vi "CRYView Model Message.vi"(8 "nData":i32, 9 "sData":string, 10 "sOption":string, 11 "sMsgData":string) -> (0 "nData_Out":i32, 1 "sData_Out":string, 3 "cView_Out":T1)   [LabVIEW 2013]
uses:
  CRYNew View Global.vi
  SubVI/CRYData View Global.vi
  CRYView Global.vi
  CRYCurveLibrary/Global/CRYCurve Library Global.vi
  CRYProject/CRYProject Editor Global.vi
panel:
  in  "Resize_Panels":bool
  out "Bar_shadow":bool
  in  "splitter_down_flag":bool=TRUE
  in  "sMsgAction":string
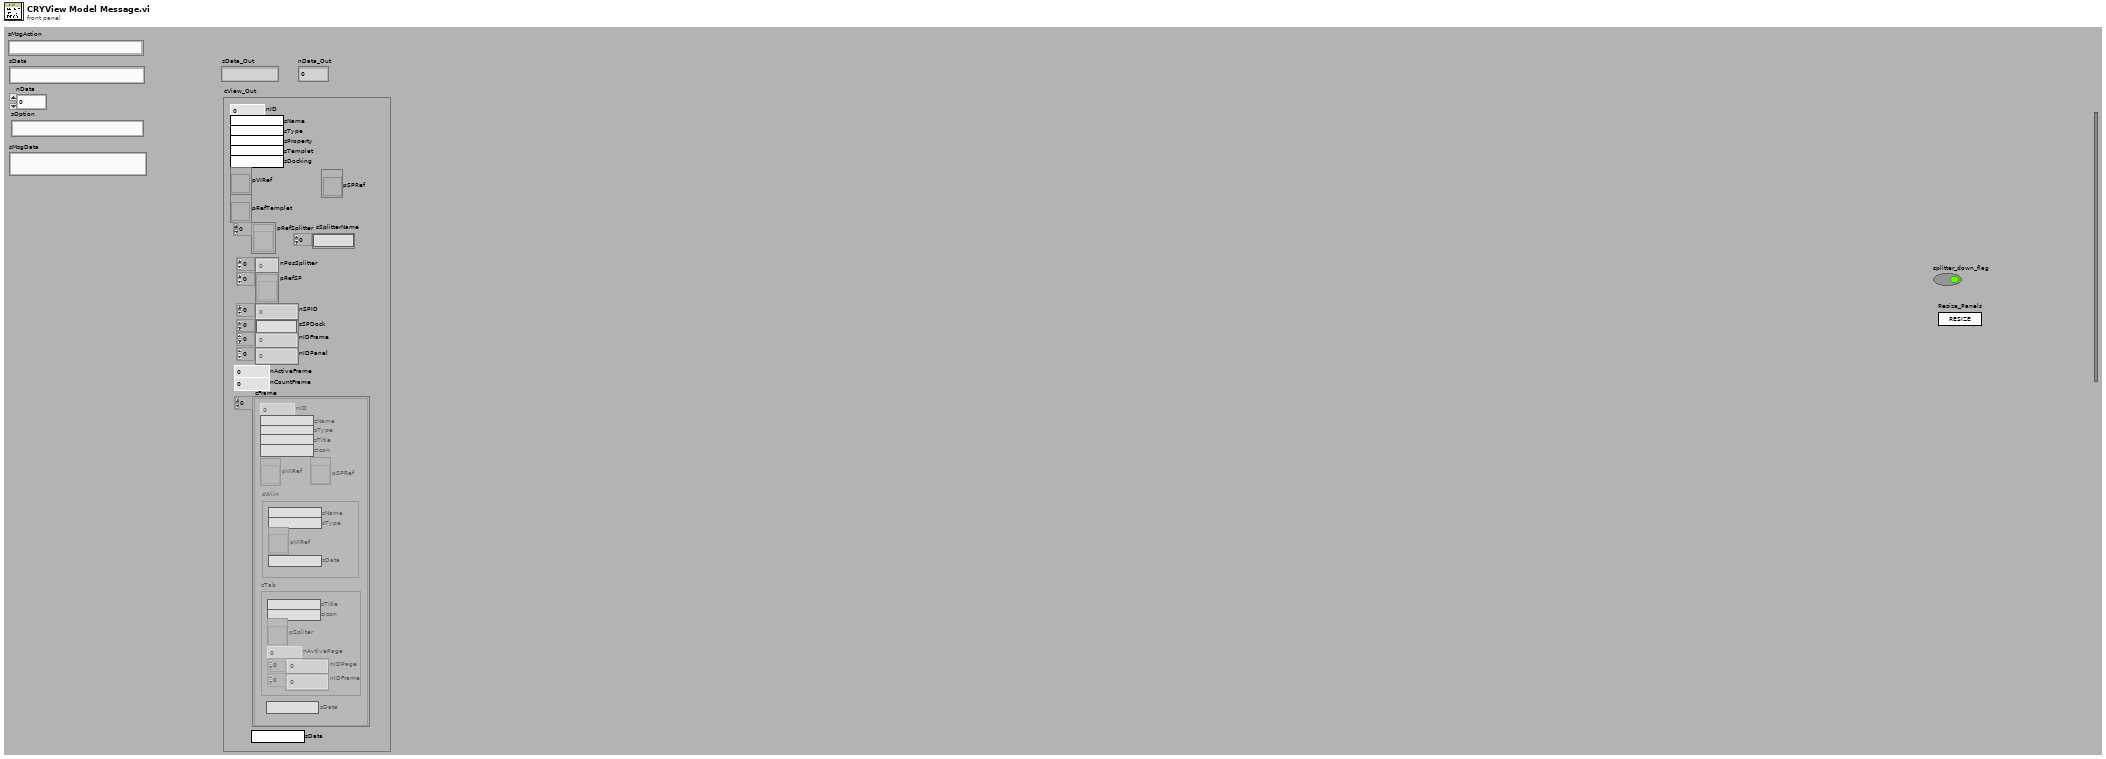
[diagram p1: front panel]
types:
  T1 = cluster{"nID":i32, "sName":string, "sType":string, "sProperty":string, "sTemplet":string, "sDocking":string, "pVIRef":refnum<vi>, "pSPRef":refnum<vi>, "pRefTemplet":refnum<vi>, "pRefSplitter":refnum<vi>[], "nPosSplitter":i32[], "pRefSP":refnum<vi>[], "nSPID":i32[], "sSPDock":string[], "nIDFrame":i32[], "nIDPanel":i32[], "nActiveFrame":i32, "nCountFrame":i32, "cFrame":cluster{"nID":i32, "sName":string, "sType":string, "sTitle":string, "sIcon":string, "pVIRef":refnum<vi>, "pSPRef":refnum<vi>, "cWiin":cluster{"sName":string, "sType":string, "pVIRef":refnum<vi>, "sData":string}, "cTab":cluster{"sTitle":string, "sIcon":string, "pSpliter":refnum<vi>, "nAvtivePage":i32, "nIDPage":i32[], "nIDFrame":i32[]}, "sData":string}[], "sData":string, "sSplitterName":string[]}
  T2 = typedef "Graph Main Info Cluster.ctl" = cluster{"Selected_BarIdx":i32, "Selected_PanelIdx":i32, "Graph Main VIRef":refnum<vi>, "ToolBarClick":bool, "Spliter Ref Array":refnum<vi>[], "Panel Ref Array":refnum<vi>[], "Spliter_matrix":i32[][], "Panel_matrix":i32[][], "child_spliterIdx_matrix":i32[][], "split_pos_matrix":i32[][], "Title State":bool, "sQueueName":string, "Frame nID":i32, "Graph VIRef Array":cluster{"Graph VIRef":refnum<vi>, "Panel Idx":i32, "Frame VIRef":refnum<vi>, "Icon Ring":i32, "Graph Type":string}[], "View Type":string}
  T3 = cluster{"Graph VIRef":refnum<vi>, "Panel Idx":i32, "Frame VIRef":refnum<vi>, "Icon Ring":i32, "Graph Type":string}[]
  T4 = cluster{"EventName":string, "Arg1":string, "Numeric":u16, "Numeric 2":u16, "AddSteps ":refnum<vi>, "Arg1 2":string, "Arg1 3":string, "Boolean":bool}
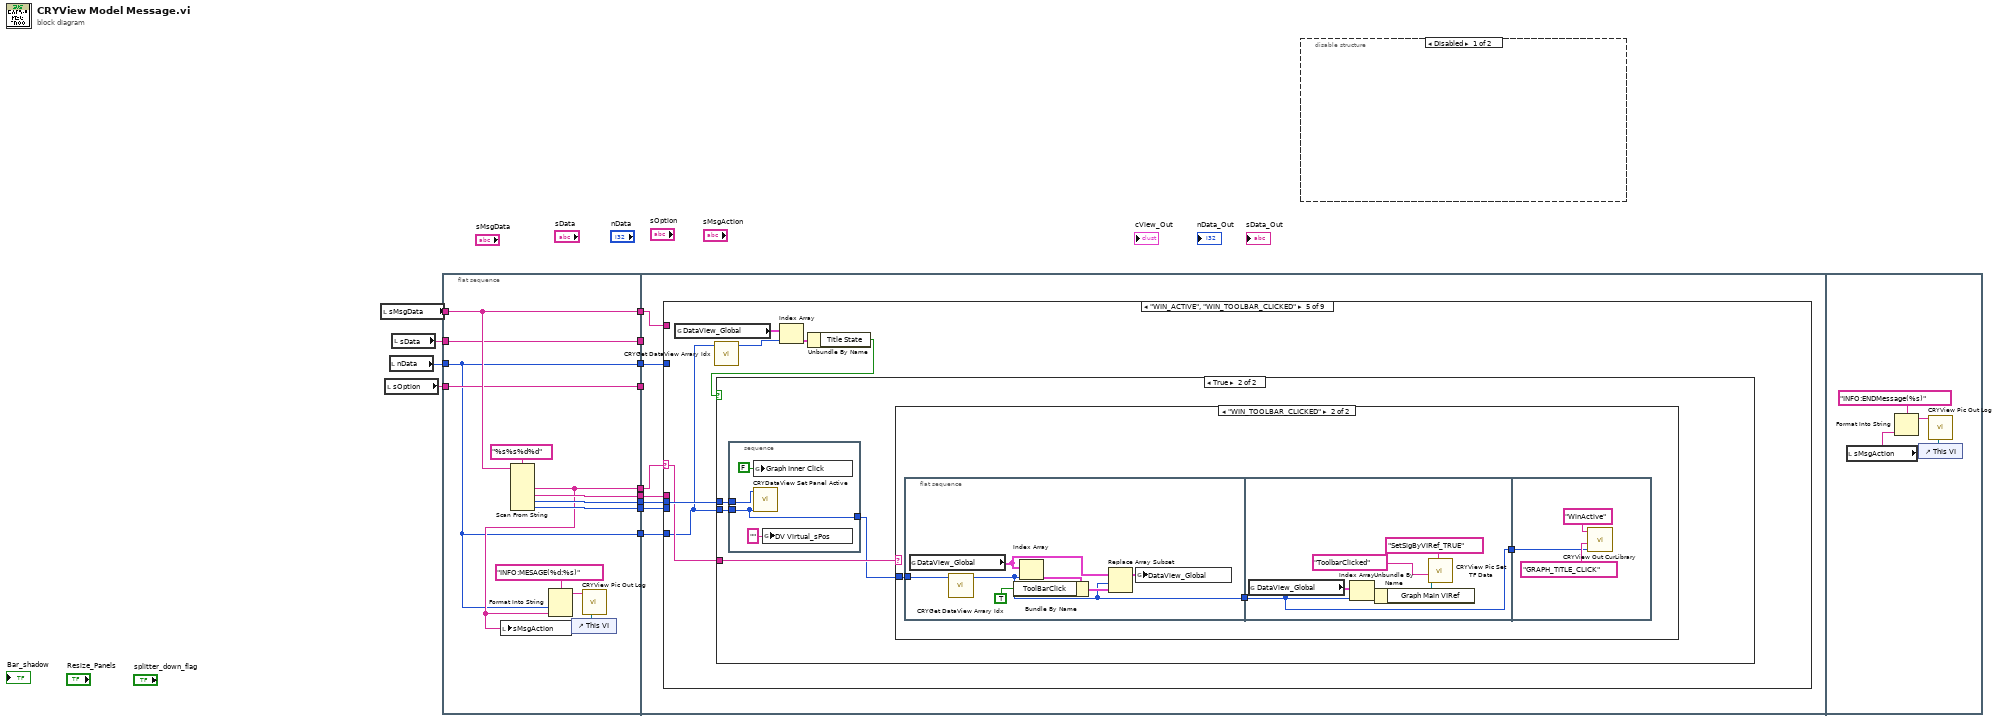
[diagram p0: block diagram]
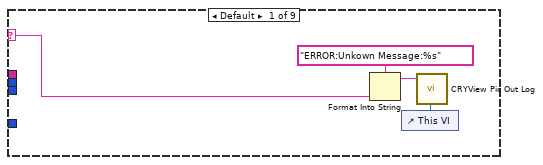
[diagram p3: hidden frame]
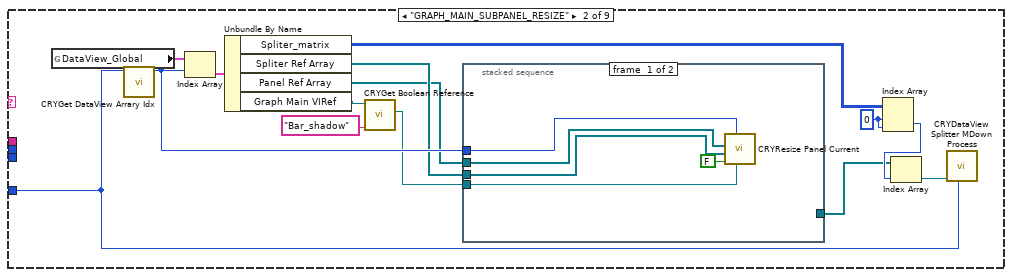
[diagram p4: hidden frame]
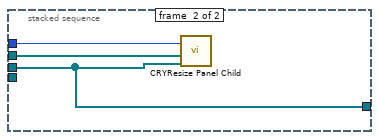
[diagram p5: hidden frame]
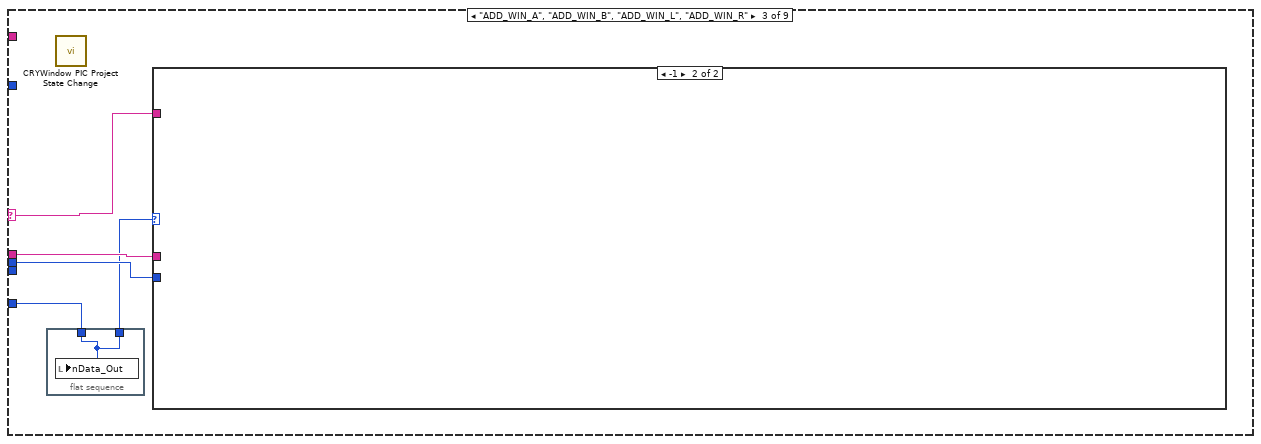
[diagram p6: hidden frame]
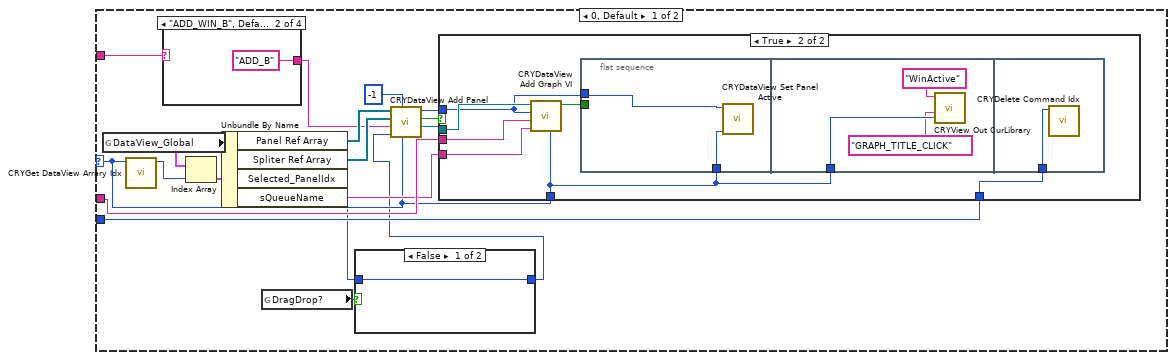
[diagram p7: hidden frame]
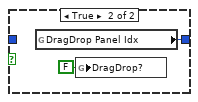
[diagram p8: hidden frame]
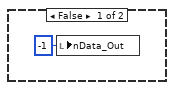
[diagram p9: hidden frame]
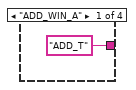
[diagram p10: hidden frame]
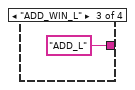
[diagram p11: hidden frame]
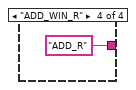
[diagram p12: hidden frame]
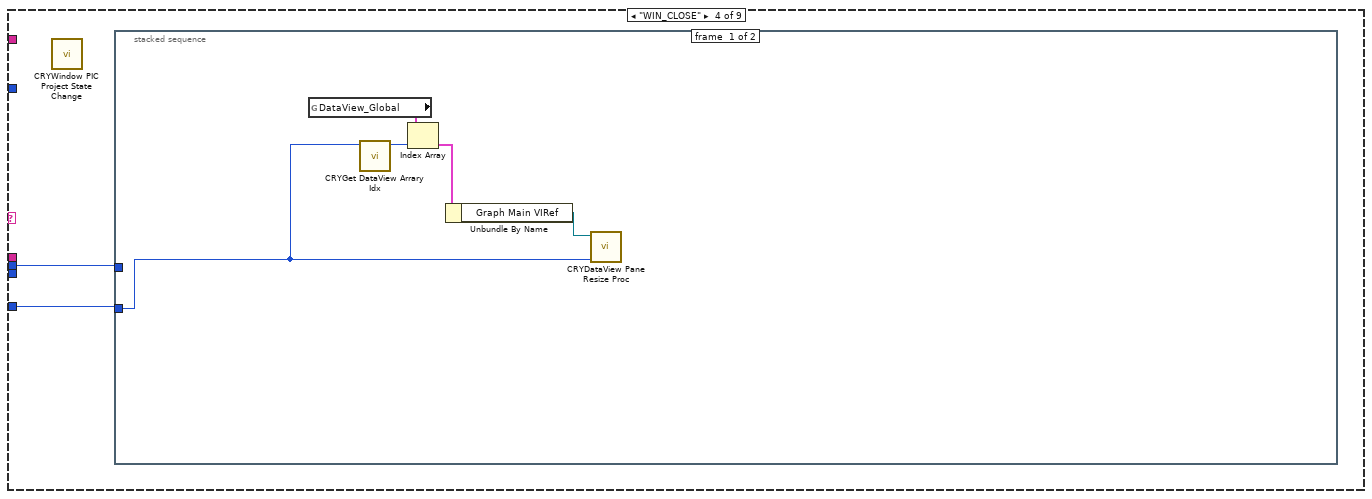
[diagram p13: hidden frame]
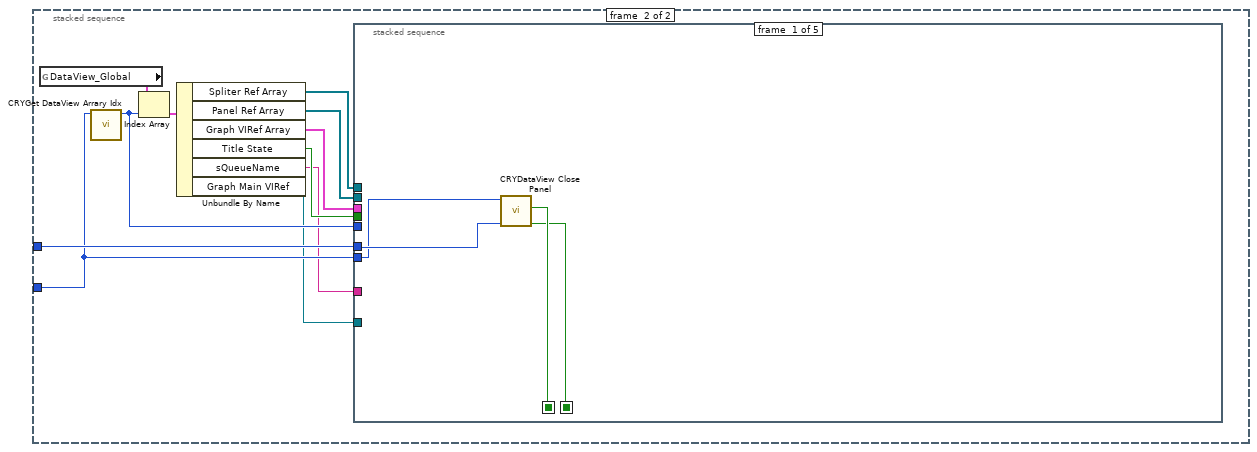
[diagram p14: hidden frame]
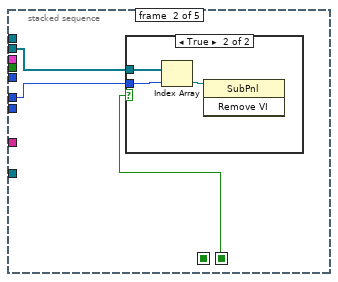
[diagram p15: hidden frame]
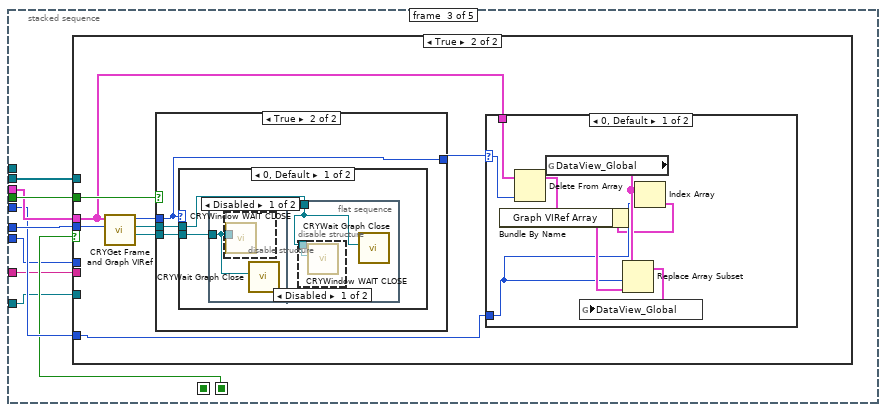
[diagram p17: hidden frame]
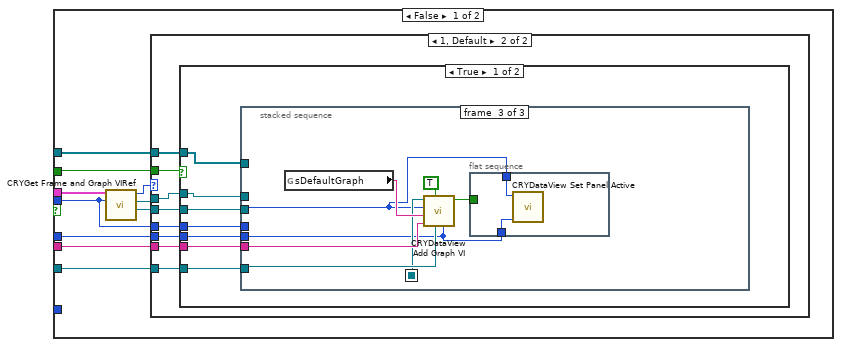
[diagram p18: hidden frame]
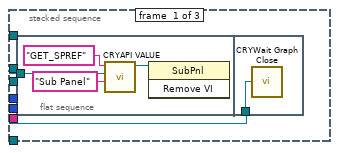
[diagram p20: hidden frame]
diagram:
  n1 = local read "sMsgData"() -> (w13:string)
  n2 = local read "sOption"() -> (w11:string)
  n3 = local read "nData"() -> (w12:i32)
  n4 = local read "sData"() -> (w5:string)
  n5 = flat-sequence {
    tunnel: w13 -> [w24]
    tunnel: w12 -> [w14]
    tunnel: w11 -> [w19]
    tunnel: [w24] -> w10
    tunnel: [w15] -> w9
    tunnel: [w23] -> w8
    tunnel: [w21] -> w7
    tunnel: [w22] -> w6
    tunnel: w5 -> [w20]
    tunnel: [w20] -> w4
    tunnel: [w14] -> w3
    tunnel: [w19] -> w2
    tunnel: [w14] -> w1
    tunnel: w10 -> [w28]
    tunnel: w9 -> [w32]
    tunnel: w8 -> [w31]
    tunnel: w7 -> [w30]
    tunnel: w6 -> [w29]
    tunnel: w4 -> [_]
    tunnel: w3 -> [w27]
    tunnel: w2 -> [_]
    tunnel: w1 -> [w26]
    frame #0 {
      n6 = Scan From String(format string="%s%s%d%d", input string=w24) -> (output 1=w15:string, output 2=w23:string, output 3=w21:i32, output 4=w22:i32)  [unwired: 2 in, 7 out]
      n7 = local write "sMsgAction"(w15) -> ()
      n8 = Format Into String(format string="INFO:MESAGE(%d:%s)", w14, w15) -> (resulting string=w17:string)  [unwired: 2 in, 1 out]
      n9 = control-ref of="This VI"() -> (w18:refnum<vi>)
      n10 = call "CRYView Pic Out Log.vi"("vi reference"=w18, "sData"=w17) -> ()  [unwired: 10 in]
    }
    frame #1 {
      n11 = case shown="\"WIN_ACTIVE\", \"WIN_TOOLBAR_CLICKED\"" w32 {
        selector: w32 -> [w34 _ w62 _ w282 _ _ w320 _]
        tunnel: w31 -> [_ _ w63 _ _ _ _ _ w328]
        tunnel: w30 -> [_ _ w61 w105 w283 _ _ w322 w332]
        tunnel: w29 -> [_ _ _ _ _ _ _ _ _]
        tunnel: w28 -> [_ _ _ _ _ _ _ w319 _]
        tunnel: w27 -> [_ _ _ _ _ _ _ _ w331]
        tunnel: w26 -> [_ w37 w60 w104 w279 _ _ w317 _]
        frame Default {
          n12 = Format Into String(format string="ERROR:Unkown Message:%s", w34) -> (resulting string=w33:string)  [unwired: 2 in, 1 out]
          n13 = control-ref of="This VI"() -> (w36:refnum<vi>)
          n14 = call "CRYView Pic Out Log.vi"("vi reference"=w36, "sData"=w33) -> ()  [unwired: 10 in]
        }
        frame "GRAPH_MAIN_SUBPANEL_RESIZE" {
          w48 = 0 ("index (row)")
          n15 = global read "CRYNew View Global.vi" "DataView_Global"() -> (w41:T2[])
          n16 = call "CRYGet DataView Arrary Idx.vi"("DataView Idx In"=w37) -> ("DataView Arrary Idx out"=w50:i32)  [unwired: 10 in]
          n17 = Index Array(array=w41, index=w50) -> (element=w42:T2)
          n18 = Unbundle By Name(w42) -> ("Spliter_matrix"=w46:i32[][], "Spliter Ref Array"=w44:refnum<vi>[], "Panel Ref Array"=w43:refnum<vi>[], "Graph Main VIRef"=w40:refnum<vi>)
          n19 = call "CRYGet Boolean Reference.vi"("Label Name"="Bar_shadow", "VI Refnum"=w40) -> ("Boolean Ref"=w38:refnum<vi>)  [unwired: 7 in, 2 out]
          n20 = stacked-sequence {
            tunnel: w44 -> [w54 w56]
            tunnel: w43 -> [w55 w58]
            tunnel: w50 -> [w53 w57]
            tunnel: [_ w56] -> w45
            tunnel: w38 -> [w52 _]
            frame #0 {
              n21 = call "CRYResize Panel Current.vi"("Bar_shadow"=w52, "DataView Array Idx"=w53, "close_panel"=FALSE, "spliter array"=w54, "SubPanel array"=w55) -> ()  [unwired: 7 in]
            }
            frame #1 {
              n22 = call "CRYResize Panel Child.vi"("spliter array"=w56, "SubPanel array"=w58, "DataView Array Idx"=w57) -> ()  [unwired: 9 in]
            }
          }
          n23 = Index Array(array=w46, index (row)=w48, index (col)=w48) -> (element=w49:i32)
          n24 = Index Array(array=w45, index=w49) -> (element=w47:refnum<vi>)
          n25 = call "CRYDataView Splitter MDown Process.vi"("DataView Index"=w37, "Selected Spliter Ref"=w47) -> ()  [unwired: 9 in, 1 out]
        }
        frame "ADD_WIN_A", "ADD_WIN_B", "ADD_WIN_L", "ADD_WIN_R" {
          n26 = flat-sequence {
            tunnel: w60 -> [w64]
            tunnel: [w64] -> w59
            frame #0 {
              n27 = local write "nData_Out"(w64) -> ()
            }
          }
          n28 = call "CRYWindow PIC Project State Change.vi"() -> ()  [unwired: 12 in]
          n29 = case shown="-1" w59 {
            selector: w59 -> [w69 _]
            tunnel: w62 -> [w79 _]
            tunnel: w63 -> [w71 _]
            tunnel: w61 -> [w68 _]
            frame 0, Default {
              n30 = global read "CRYNew View Global.vi" "DataView_Global"() -> (w82:T2[])
              n31 = call "CRYGet DataView Arrary Idx.vi"("DataView Idx In"=w69) -> ("DataView Arrary Idx out"=w81:i32)  [unwired: 10 in]
              n32 = case shown="\"ADD_WIN_B\", Default" w79 {
                tunnel: ["ADD_T" ("input 1") "ADD_B" ("input 1") "ADD_L" ("input 1") "ADD_R" ("input 1")] -> w75
                frame "ADD_WIN_A" {
                }
                frame "ADD_WIN_B", Default {
                }
                frame "ADD_WIN_L" {
                }
                frame "ADD_WIN_R" {
                }
              }
              n33 = Index Array(array=w82, index=w81) -> (element=w80:T2)
              n34 = Unbundle By Name(w80) -> ("Panel Ref Array"=w77:refnum<vi>[], "Spliter Ref Array"=w76:refnum<vi>[], "Selected_PanelIdx"=w66:i32, "sQueueName"=w70:string)
              n35 = global read "CRYData View Global.vi" "DragDrop?"() -> (w67:bool)
              n36 = case shown="False" w67 {
                tunnel: [w83 w84] -> w65
                tunnel: w66 -> [w83 _]
                frame False {
                }
                frame True {
                  n37 = global read "CRYData View Global.vi" "DragDrop Panel Idx"() -> (w84:i32)
                  n38 = global write "CRYData View Global.vi" "DragDrop?"(FALSE ("DragDrop?")) -> ()
                }
              }
              n39 = call "CRYDataView Add Panel.vi"("DataView Index"=w69, "panel_index"=-1, "Selected Panel Idx"=w65, "SAdd_Pos"=w75, "spliter array"=w76, "SubPanel array"=w77) -> ("Panel Ref"=w72:refnum<vi>, "bResult"=w74:bool, "panel_index_out"=w73:i32)  [unwired: 3 in]
              n40 = case shown="True" w74 {
                tunnel: w73 -> [_ w90]
                tunnel: w72 -> [_ w93]
                tunnel: w71 -> [_ w92]
                tunnel: w70 -> [_ w91]
                tunnel: w68 -> [_ w88]
                tunnel: w69 -> [_ w87]
                frame False {
                  n41 = local write "nData_Out"(-1 ("nData_Out")) -> ()
                }
                frame True {
                  n42 = call "CRYDataView Add Graph VI.vi"("DataView Idx"=w87, "Queue Name"=w91, "GraphType"=w92, "panel_index"=w90, "Panel Ref In"=w93) -> ("bResult"=w89:bool)  [unwired: 6 in]
                  n43 = flat-sequence {
                    tunnel: w90 -> [w95]
                    tunnel: w89 -> [_]
                    tunnel: w87 -> [w94]
                    tunnel: w87 -> [w98]
                    tunnel: w88 -> [w99]
                    frame #0 {
                      n44 = call "CRYDataView Set Panel Active.vi"("DataView Index"=w94, "Selected Panel Idx In"=w95) -> ()  [unwired: 10 in]
                    }
                    frame #1 {
                      n45 = call "CRYView Out CurLibrary.vi"("DataView Idx"=w98, "sData"="GRAPH_TITLE_CLICK", "sAction"="WinActive") -> ()  [unwired: 7 in, 2 out]
                    }
                    frame #2 {
                      n46 = call "CRYDelete Command Idx.vi"("Command Idx In"=w99) -> ()  [unwired: 11 in]
                    }
                  }
                }
              }
            }
            frame -1 {
            }
          }
        }
        frame "WIN_CLOSE" {
          n47 = call "CRYWindow PIC Project State Change.vi"() -> ()  [unwired: 12 in]
          n48 = stacked-sequence {
            tunnel: w105 -> [_ w121]
            tunnel: w104 -> [w110 w120]
            frame #0 {
              n49 = global read "CRYNew View Global.vi" "DataView_Global"() -> (w109:T2[])
              n50 = call "CRYGet DataView Arrary Idx.vi"("DataView Idx In"=w110) -> ("DataView Arrary Idx out"=w108:i32)  [unwired: 10 in]
              n51 = Index Array(array=w109, index=w108) -> (element=w107:T2)
              n52 = Unbundle By Name(w107) -> ("Graph Main VIRef"=w106:refnum<vi>)
              n53 = call "CRYDataView Pane Resize Proc.vi"("DataView Index"=w110, "VI Ref"=w106) -> ()  [unwired: 10 in]
            }
            frame #1 {
              n54 = global read "CRYNew View Global.vi" "DataView_Global"() -> (w119:T2[])
              n55 = call "CRYGet DataView Arrary Idx.vi"("DataView Idx In"=w120) -> ("DataView Arrary Idx out"=w118:i32)  [unwired: 10 in]
              n56 = Index Array(array=w119, index=w118) -> (element=w113:T2)
              n57 = Unbundle By Name(w113) -> ("Spliter Ref Array"=w117:refnum<vi>[], "Panel Ref Array"=w116:refnum<vi>[], "Graph VIRef Array"=w115:T3, "Title State"=w114:bool, "sQueueName"=w112:string, "Graph Main VIRef"=w111:refnum<vi>)
              n58 = stacked-sequence {
                seq-local: [w125 _ _ _ _] -> [_ _ _ w242 _]
                seq-local: [w123 _ _ _ _] -> [_ w128 w136 _ _]
                tunnel: w121 -> [w124 w126 w140 _ w262]
                tunnel: w120 -> [w122 _ w133 w240 w270]
                tunnel: w116 -> [_ w127 w132 w243 _]
                tunnel: w117 -> [_ _ _ w239 _]
                tunnel: w118 -> [_ _ w137 w241 w260]
                tunnel: w115 -> [_ _ w138 _ _]
                tunnel: w114 -> [_ _ w139 _ _]
                tunnel: w112 -> [_ _ w135 _ _]
                tunnel: w111 -> [_ _ w134 _ _]
                frame #0 {
                  n59 = call "CRYDataView Close Panel.vi"("Panel_Idx"=w124, "DataView Index"=w122) -> ("bResult"=w123:bool, "bHaveChild"=w125:bool)  [unwired: 7 in, 1 out]
                }
                frame #1 {
                  n60 = case shown="True" w128 {
                    tunnel: w127 -> [_ w131]
                    tunnel: w126 -> [_ w130]
                    frame False {
                    }
                    frame True {
                      n61 = Index Array(array=w131, index=w130) -> (element=w129:refnum<vi>)
                      n62 = invoke class="SubPnl" method="Remove VI"(reference=w129) -> ()  [unwired: 2 in, 3 out]
                    }
                  }
                }
                frame #2 {
                  n63 = case shown="True" w136 {
                    tunnel: w140 -> [w145 w217]
                    tunnel: w139 -> [w150 w216]
                    tunnel: w138 -> [w149 w211]
                    tunnel: w137 -> [_ w210]
                    tunnel: w135 -> [w146 _]
                    tunnel: w134 -> [w144 _]
                    tunnel: w133 -> [w143 _]
                    tunnel: w132 -> [w142 _]
                    frame False {
                      n64 = call "CRYGet Frame and Graph VIRef.vi"("Panel Idx"=w145, "Graph VIRef Array"=w149) -> ("Graph VIRef"=w148:refnum<vi>, "Frame VIRef"=w147:refnum<vi>, "Graph VIRef Array Index"=w141:i32)  [unwired: 5 in, 2 out]
                      n65 = case shown="1, Default" w141 {
                        tunnel: w150 -> [_ w158]
                        tunnel: w148 -> [_ w157]
                        tunnel: w147 -> [_ w156]
                        tunnel: w146 -> [_ w155]
                        tunnel: w145 -> [_ w154]
                        tunnel: w144 -> [_ w153]
                        tunnel: w143 -> [_ w152]
                        tunnel: w142 -> [_ w151]
                        frame -1 {
                        }
                        frame 1, Default {
                          n66 = case shown="True" w158 {
                            tunnel: w157 -> [w164 w197]
                            tunnel: w156 -> [w165 _]
                            tunnel: w155 -> [w163 w196]
                            tunnel: w154 -> [w162 w195]
                            tunnel: w153 -> [w161 w194]
                            tunnel: w152 -> [w160 w193]
                            tunnel: w151 -> [w159 w192]
                            frame True {
                              n67 = stacked-sequence {
                                seq-local: [_ w173 _] -> [_ _ w185]
                                tunnel: w165 -> [w167 w174 _]
                                tunnel: w164 -> [w166 _ _]
                                tunnel: w163 -> [_ _ w188]
                                tunnel: w162 -> [_ w175 w182]
                                tunnel: w161 -> [_ _ w187]
                                tunnel: w160 -> [_ _ w183]
                                tunnel: w159 -> [_ w176 _]
                                frame #0 {
                                n68 = flat-sequence {
                                tunnel: w167 -> [w169]
                                tunnel: w166 -> [w172]
                                frame #0 {
                                n69 = call "CRYAPI VALUE.vi"("sControlName"="Sub Panel", "pVIRef"=w169, "sAction"="GET_SPREF") -> ("pSPRef"=w168:refnum<vi>)  [unwired: 2 in, 6 out]
                                n70 = invoke class="SubPnl" method="Remove VI"(reference=w168) -> ()  [unwired: 2 in, 3 out]
                                }
                                frame #1 {
                                n71 = call "CRYWait Graph Close.vi"("vi reference"=w172) -> ()  [unwired: 11 in]
                                }
                                }
                                }
                                frame #1 {
                                n72 = flat-sequence {
                                tunnel: w176 -> [w180]
                                tunnel: w175 -> [w179]
                                tunnel: [w177] -> w173
                                tunnel: w174 -> [w181]
                                frame #0 {
                                n73 = Index Array(array=w180, index=w179) -> (element=w178:refnum<vi>)
                                n74 = invoke class="SubPnl" method="Remove VI"(reference=w178) -> (reference out=w177:refnum<vi>)  [unwired: 2 in, 2 out]
                                }
                                frame #1 {
                                n75 = call "CRYWait Graph Close.vi"("vi reference"=w181) -> ()  [unwired: 11 in]
                                }
                                }
                                }
                                frame #2 {
                                n76 = global read "CRYView Global.vi" "sDefaultGraph"() -> (w189:string)
                                n77 = call "CRYDataView Add Graph VI.vi"("DataView Idx"=w183, "Graph Main VIRef In"=w187, "isFirstPanel"=TRUE, "Queue Name"=w188, "GraphType"=w189, "panel_index"=w182, "Panel Ref In"=w185) -> ("bResult"=w184:bool)  [unwired: 4 in]
                                n78 = flat-sequence {
                                tunnel: w183 -> [w191]
                                tunnel: w184 -> [_]
                                tunnel: w182 -> [w190]
                                frame #0 {
                                n79 = call "CRYDataView Set Panel Active.vi"("DataView Index"=w191, "Selected Panel Idx In"=w190) -> ()  [unwired: 10 in]
                                }
                                }
                                }
                              }
                            }
                            frame False {
                              n80 = stacked-sequence {
                                seq-local: [w201 _ _] -> [_ _ w203]
                                tunnel: w197 -> [_ w202 _]
                                tunnel: w196 -> [_ _ w208]
                                tunnel: w195 -> [w199 _ w207]
                                tunnel: w194 -> [_ _ w206]
                                tunnel: w193 -> [_ _ w204]
                                tunnel: w192 -> [w200 _ _]
                                frame #0 {
                                n81 = Index Array(array=w200, index=w199) -> (element=w198:refnum<vi>)
                                n82 = invoke class="SubPnl" method="Remove VI"(reference=w198) -> (reference out=w201:refnum<vi>)  [unwired: 2 in, 2 out]
                                }
                                frame #1 {
                                n83 = call "CRYWait Graph Close.vi"("vi reference"=w202) -> ()  [unwired: 11 in]
                                }
                                frame #2 {
                                n84 = global read "CRYView Global.vi" "sDefaultGraph"() -> (w209:string)
                                n85 = call "CRYDataView Add Graph VI.vi"("DataView Idx"=w204, "Graph Main VIRef In"=w206, "isFirstPanel"=TRUE, "Queue Name"=w208, "GraphType"=w209, "panel_index"=w207, "Panel Ref In"=w203) -> ()  [unwired: 4 in, 1 out]
                                }
                              }
                            }
                          }
                        }
                      }
                    }
                    frame True {
                      n86 = call "CRYGet Frame and Graph VIRef.vi"("Panel Idx"=w217, "Graph VIRef Array"=w211) -> ("Graph VIRef"=w213:refnum<vi>, "Frame VIRef"=w214:refnum<vi>, "Graph VIRef Array Index"=w215:i32)  [unwired: 5 in, 2 out]
                      n87 = case shown="True" w216 {
                        tunnel: w215 -> [w226 w230]
                        tunnel: w214 -> [_ w231]
                        tunnel: w213 -> [w227 w232]
                        tunnel: [w226 w230] -> w212
                        frame False {
                          n88 = case shown="0, Default" w226 {
                            tunnel: w227 -> [w228 _]
                            frame 0, Default {
                              n89 = disable-structure shown="Disabled" {
                                disable-tunnel: w228 -> [w229 _]
                                frame Disabled {
                                n90 = call "CRYWindow WAIT CLOSE.vi"("vi reference"=w229) -> ()  [unwired: 11 in]
                                }
                                frame Enabled {
                                }
                              }
                              n91 = call "CRYWait Graph Close.vi"("vi reference"=w228) -> ()  [unwired: 11 in]
                            }
                            frame -1 {
                            }
                          }
                        }
                        frame True {
                          n92 = case shown="0, Default" w230 {
                            tunnel: w232 -> [w234 _]
                            tunnel: w231 -> [w233 _]
                            frame 0, Default {
                              n93 = flat-sequence {
                                tunnel: w234 -> [w235]
                                tunnel: w233 -> [w237]
                                frame #0 {
                                n94 = disable-structure shown="Disabled" {
                                disable-tunnel: w235 -> [w236 _]
                                frame Disabled {
                                n95 = call "CRYWindow WAIT CLOSE.vi"("vi reference"=w236) -> ()  [unwired: 11 in]
                                }
                                frame Enabled {
                                }
                                }
                                n96 = call "CRYWait Graph Close.vi"("vi reference"=w235) -> ()  [unwired: 11 in]
                                }
                                frame #1 {
                                n97 = disable-structure shown="Disabled" {
                                disable-tunnel: w237 -> [w238 _]
                                frame Disabled {
                                n98 = call "CRYWindow WAIT CLOSE.vi"("vi reference"=w238) -> ()  [unwired: 11 in]
                                }
                                frame Enabled {
                                }
                                }
                                n99 = call "CRYWait Graph Close.vi"("vi reference"=w237) -> ()  [unwired: 11 in]
                                }
                              }
                            }
                            frame -1 {
                            }
                          }
                        }
                      }
                      n100 = case shown="0, Default" w212 {
                        selector: w212 -> [w224 _]
                        tunnel: w211 -> [w225 _]
                        tunnel: w210 -> [w219 _]
                        frame 0, Default {
                          n101 = Delete From Array(array=w225, index=w224) -> (array with subset deleted=w223:T3)  [unwired: 1 in, 1 out]
                          n102 = global read "CRYNew View Global.vi" "DataView_Global"() -> (w220:T2[])
                          n103 = Index Array(array=w220, index=w219) -> (element=w218:T2)
                          n104 = Bundle By Name(cluster=w218, "Graph VIRef Array"=w223) -> (w222:T2)
                          n105 = Replace Array Subset(array=w220, new element=w222, index=w219) -> (w221:T2[])
                          n106 = global write "CRYNew View Global.vi" "DataView_Global"(w221) -> ()
                        }
                        frame -1 {
                        }
                      }
                    }
                  }
                }
                frame #3 {
                  n107 = case shown="True" w242 {
                    tunnel: w243 -> [_ w248]
                    tunnel: w239 -> [_ w247]
                    tunnel: w241 -> [_ w246]
                    tunnel: w240 -> [w244 w245]
                    tunnel: [w244 w245] -> _
                    frame False {
                    }
                    frame True {
                      n108 = flat-sequence {
                        tunnel: w248 -> [w253]
                        tunnel: w247 -> [w252]
                        tunnel: w246 -> [w254]
                        tunnel: [w254] -> w251
                        tunnel: [w253] -> w250
                        tunnel: [w252] -> w249
                        tunnel: w251 -> [w258]
                        tunnel: w250 -> [w257]
                        tunnel: w249 -> [w256]
                        frame #0 {
                          n109 = call "CRYResize Panel Current.vi"("DataView Array Idx"=w254, "close_panel"=TRUE, "spliter array"=w252, "SubPanel array"=w253) -> ()  [unwired: 8 in]
                        }
                        frame #1 {
                          n110 = call "CRYResize Panel Child.vi"("spliter array"=w256, "SubPanel array"=w257, "DataView Array Idx"=w258) -> ()  [unwired: 9 in]
                        }
                      }
                    }
                  }
                }
                frame #4 {
                  # "if delete no actived graph, preview actived Panel index\nif deleted, first index."
                  n111 = global read "CRYNew View Global.vi" "DataView_Global"() -> (w269:T2[])
                  n112 = Index Array(array=w269, index=w260) -> (element=w268:T2)
                  n113 = Unbundle By Name(w268) -> ("Panel_matrix"=w267:i32[][], "Selected_PanelIdx"=w263:i32)
                  n114 = Index Array(array=w267, index (row)=1, index (col)=0) -> (element=w264:i32)
                  n115 = Equal?(x=w263, y=w262) -> (x = y?=w261:bool)
                  n116 = case shown="False" w261 {
                    tunnel: w270 -> [_ w276]
                    tunnel: w264 -> [w274 w275]
                    tunnel: [w274 w275] -> w259
                    frame False {
                    }
                    frame True {
                      n117 = call "CRYDataView Set Panel Active.vi"("DataView Index"=w276, "Selected Panel Idx In"=w275) -> ()  [unwired: 10 in]
                    }
                  }
                  n118 = flat-sequence {
                    tunnel: w260 -> [w271]
                    tunnel: w259 -> [_]
                    frame #0 {
                      n119 = call "CRYView Out CurLibrary.vi"("DataView Idx"=w271, "sData"="GRAPH_TITLE_CLICK", "sAction"="WinActive") -> ()  [unwired: 7 in, 2 out]
                    }
                  }
                }
              }
            }
          }
        }
        frame "WIN_ACTIVE", "WIN_TOOLBAR_CLICKED" {
          n120 = global read "CRYNew View Global.vi" "DataView_Global"() -> (w281:T2[])
          n121 = call "CRYGet DataView Arrary Idx.vi"("DataView Idx In"=w279) -> ("DataView Arrary Idx out"=w280:i32)  [unwired: 10 in]
          n122 = Index Array(array=w281, index=w280) -> (element=w278:T2)
          n123 = Unbundle By Name(w278) -> ("Title State"=w277:bool)
          n124 = case shown="True" w277 {
            tunnel: w283 -> [w285 w293]
            tunnel: w282 -> [_ w292]
            tunnel: w279 -> [w284 w290]
            frame False {
              n125 = stacked-sequence {
                tunnel: w285 -> [w288]
                tunnel: w284 -> [w287]
                frame #0 {
                  n126 = global write "CRYCurve Library Global.vi" "Graph Inner Click"(FALSE ("Graph Inner Click")) -> ()
                  n127 = call "CRYDataView Set Panel Active.vi"("DataView Index"=w287, "Selected Panel Idx In"=w288) -> ()  [unwired: 10 in]
                  n128 = global write "CRYNew View Global.vi" "DV Virtual_sPos"("" ("DV Virtual_sPos")) -> ()
                }
              }
            }
            frame True {
              n129 = stacked-sequence {
                tunnel: w293 -> [w315]
                tunnel: w290 -> [w314]
                tunnel: [w314] -> w291
                frame #0 {
                  n130 = global write "CRYCurve Library Global.vi" "Graph Inner Click"(FALSE ("Graph Inner Click")) -> ()
                  n131 = call "CRYDataView Set Panel Active.vi"("DataView Index"=w314, "Selected Panel Idx In"=w315) -> ()  [unwired: 10 in]
                  n132 = global write "CRYNew View Global.vi" "DV Virtual_sPos"("" ("DV Virtual_sPos")) -> ()
                }
              }
              n133 = case shown="\"WIN_TOOLBAR_CLICKED\"" w292 {
                tunnel: w291 -> [_ w296]
                frame "False", Default {
                }
                frame "WIN_TOOLBAR_CLICKED" {
                  n134 = flat-sequence {
                    tunnel: w296 -> [w298]
                    tunnel: [w297] -> w295
                    tunnel: w295 -> [w304]
                    tunnel: [w304] -> w294
                    tunnel: w294 -> [w310]
                    frame #0 {
                      n135 = global read "CRYNew View Global.vi" "DataView_Global"() -> (w301:T2[])
                      n136 = call "CRYGet DataView Arrary Idx.vi"("DataView Idx In"=w298) -> ("DataView Arrary Idx out"=w297:i32)  [unwired: 10 in]
                      n137 = Index Array(array=w301, index=w297) -> (element=w300:T2)
                      n138 = Bundle By Name(cluster=w300, "ToolBarClick"=TRUE) -> (w302:T2)
                      n139 = Replace Array Subset(array=w301, new element=w302, index=w297) -> (w299:T2[])
                      n140 = global write "CRYNew View Global.vi" "DataView_Global"(w299) -> ()
                    }
                    frame #1 {
                      n141 = global read "CRYNew View Global.vi" "DataView_Global"() -> (w309:T2[])
                      n142 = Index Array(array=w309, index=w304) -> (element=w308:T2)
                      n143 = Unbundle By Name(w308) -> ("Graph Main VIRef"=w305:refnum<vi>)
                      n144 = call "CRYView Pic Set TF Data.vi"("sAction"="SetSigByVIRef_TRUE", "pVIRef"=w305, "sData"="ToolbarClicked") -> ()  [unwired: 9 in]
                    }
                    frame #2 {
                      n145 = call "CRYView Out CurLibrary.vi"("DataView Idx"=w310, "sData"="GRAPH_TITLE_CLICK", "sAction"="WinActive") -> ()  [unwired: 7 in, 2 out]
                    }
                  }
                }
              }
            }
          }
        }
        frame "DOCKING" {
          n146 = call "CRYWindow PIC Project State Change.vi"() -> ()  [unwired: 12 in]
        }
        frame "WIN_MOUSE_MOVE" {
        }
        frame "CURSOR_VIEW", "DA_AXIS_PHASE", "DA_CUR_HIDE", "DA_CUR_PRO", "DA_CUR_VIEW", "DA_LEG_HIDE", "DA_LEG_VIEW", "DA_PRE_HIDE", "DA_PRE_VIEW", "DA_PROPERTY", "DROP", "LEGEND_VIEW", "PREVIEW_VIEW", "X_AUTOSCALE", "Y1_AUTOSCALE", "Y2_AUTOSCALE" {
          n147 = call "CRYWindow PIC Project State Change.vi"() -> ()  [unwired: 12 in]
          n148 = case shown="\"DROP\"" w320 {
            tunnel: [w324 w326] -> w321
            tunnel: w322 -> [_ _]
            tunnel: w319 -> [w325 w327]
            tunnel: [w325 w327] -> w318
            tunnel: w317 -> [w324 w326]
            frame "DROP" {
            }
            frame Default {
            }
          }
          n149 = call "CRYView Out CurLibrary.vi"("DataView Idx"=w321, "sData"=w318, "sAction"="OnlyNeedVIRef") -> ()  [unwired: 7 in, 2 out]
        }
        frame "ADD_DOC" {
          n150 = Number To Decimal String(number=w331) -> (decimal integer string=w330:string)  [unwired: 1 in]
          n151 = Number To Decimal String(number=w332) -> (decimal integer string=w329:string)  [unwired: 1 in]
          n152 = global read "CRYProject Editor Global.vi" "cMsgProject"() -> (w335:T4)
          n153 = Bundle By Name(cluster=w335, "EventName"="ADD_DOC", "Arg1"=w330, "Arg1 2"=w328, "Arg1 3"=w329) -> (w333:T4)
          n154 = call "CRYPIC PUSH Message to MainMenu.vi"("cMsgProject"=w333) -> ()  [unwired: 11 in]
        }
      }
    }
    frame #2 {
      n155 = local read "sMsgAction"() -> (w336:string)
      n156 = Format Into String(format string="INFO:ENDMessage(%s)", w336) -> (resulting string=w338:string)  [unwired: 2 in, 1 out]
      n157 = control-ref of="This VI"() -> (w339:refnum<vi>)
      n158 = call "CRYView Pic Out Log.vi"("vi reference"=w339, "sData"=w338) -> ()  [unwired: 10 in]
    }
  }
  n159 = disable-structure shown="Disabled" {
    frame Disabled {
    }
    frame Enabled {
    }
  }
